vi "createUnitsAttribute.vi"(8 "error in (no error)":errorcluster, 10 "Variant":variant, 11 "WriteAttribute in":refnum<class "XMLAttributeGenerator.lvclass">) -> (0 "error out":errorcluster, 2 "AttributeString":string, 3 "WriteAttribute out":refnum<class "XMLAttributeGenerator.lvclass">)   [LabVIEW 2016, in "XML.lvlib" / "XMLAttributeGenerator.lvclass"]
doc: "This method creates a unit attribute for XML generation based on the input data type."
uses:
  <userlib>/Common/XML/XMLAttributeGenerator/XMLAttributeGenerator.lvclass
  <userlib>/Common/XML/Typedefs/AttributeElements.ctl
  <userlib>/Common/XML/XMLAttributeGenerator/formatAttributeString.vi
  <vilib>/dlg_ctls.llb/Space Constant.vi
  <vilib>/Utility/VariantDataType/VariantType.lvlib
  <userlib>/Common/XML/XML.lvlib
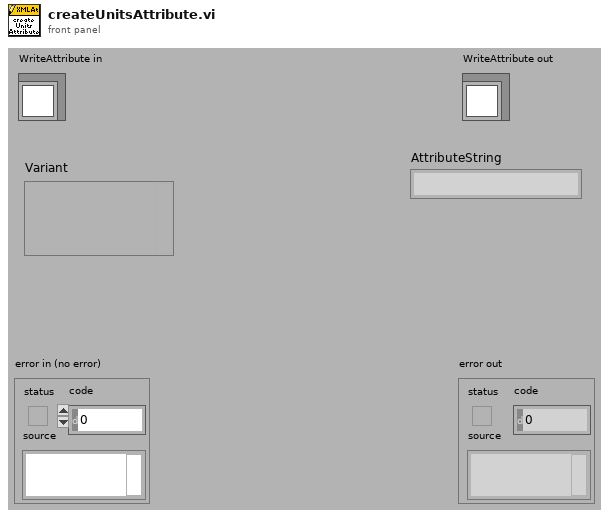
[diagram p1: front panel]
types:
  T1 = typedef "XML.lvlib/AttributeElements.ctl" = cluster{"attributeType":string, "attributeValue":string}
  T2 = typedef "LVNumericRepresentation.ctl" = enum32{"Extended Precision", "Double Precision", "Single Precision", "Long", "Word", "Byte", "Unsigned Long", "Unsigned Word", "Unsigned Byte", "Complex Extended", "Complex Double", "Complex Single", "Quad", "Unsigned Quad", "Fixed-Point"}
  T3 = typedef "VariantType.lvlib/UnitInfo.ctl" = cluster{"UnitType":T4, "Exponent":i16}
  T4 = typedef "VariantType.lvlib/UnitType.ctl" = enum16{"Radians", "Steradians", "Seconds", "Meters", "Kilograms", "Amperes", "Kelvins", "Moles", "Candelas", "InvalidUnit"}
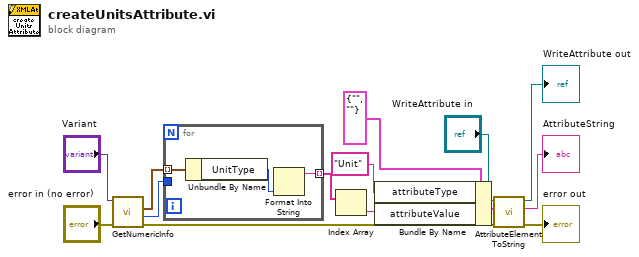
[diagram p0: block diagram]
diagram:
  n1 = call <vilib>:"GetNumericInfo.vi"("error in (no error)"="error in (no error)", "Variant"="Variant") -> ("error out"=w2:errorcluster, "representation"=w11:T2, "Units"=w13:T3[])  [unwired: 6 in, 1 out]
  n2 = for {
    tunnel: w13 -> [w17] mode=indexing
    tunnel: [w15] -> w9 mode=indexing
    tunnel: w11 -> [_]
    n3 = Unbundle By Name(w17) -> ("UnitType"=w16:T4)
    n4 = Format Into String(w16) -> (resulting string=w15:string)  [unwired: 3 in, 1 out]
  }
  n5 = Index Array(array=w9) -> (element=w8:string)  [unwired: 1 in]
  n6 = Bundle By Name(cluster=T1 {"attributeType"="", "attributeValue"=""} ("attributeData 2"), "attributeType"="Unit", "attributeValue"=w8) -> (w7:T1)
  n7 = call <userlib>:"AttributeElementToString.vi"("error in (no error)"=w2, "attributeElement"=w7, "WriteAttribute in"="WriteAttribute in") -> ("error out"=→"error out":errorcluster, "AttributeString"=→"AttributeString":string, "WriteAttribute out"=→"WriteAttribute out":refnum<class "XMLAttributeGenerator.lvclass">)  [unwired: 6 in]
